vi "CLD3 FGV Timer Exercise.vi"(8 "Error In":errorcluster, 10 "Time Target (s)":dbl, 11 "Timer Mode":T1) -> (0 "Error Out":errorcluster, 3 "Elapsed Time (s.ss)":dbl)   [LabVIEW 2009]
doc: "CLD 3 Exercise"
uses:
  CLD3 FGV Mode.ctl
panel:
  out "Has Time Elapsed":bool
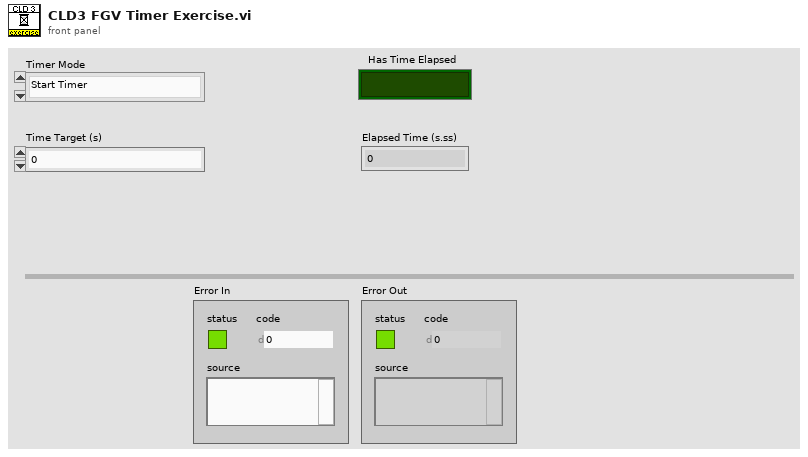
[diagram p1: front panel]
types:
  T1 = typedef "CLD3 FGV Mode.ctl" = enum16{"Start Timer", "Read Time", "Pause", "Resume"}
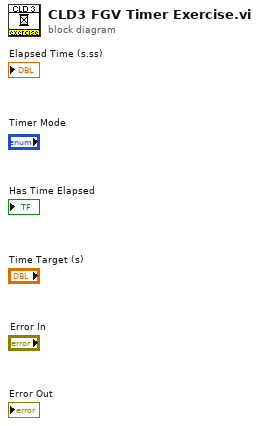
[diagram p0: block diagram]
diagram:
